vi "Test Initialize.vi"(0 "niDTS BT Rx Test in":refnum<class "niDTS BT Rx Test.lvclass">, 11 "error in (no error)":errorcluster) -> (4 "niDTS BT Rx Test out":refnum<class "niDTS BT Rx Test.lvclass">, 15 "error out":errorcluster)   [LabVIEW 2015, in "niDTS BT.lvlib" / "niDTS BT Rx Test.lvclass"]
uses:
  niDTS BT Rx Test.lvclass
  TestStand/TestStep/Objects/niDTS TestStep.lvclass
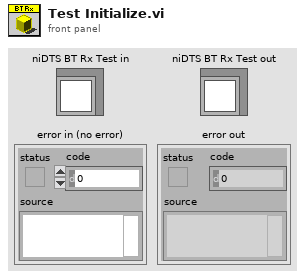
[diagram p1: front panel]
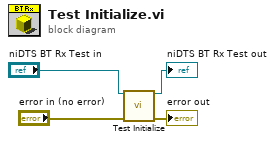
[diagram p0: block diagram]
diagram:
  n1 = call-parent "Test Initialize.vi"("niDTS TestStep in"="niDTS BT Rx Test in", "error in (no error)"="error in (no error)") -> ("niDTS TestStep out"=→"niDTS BT Rx Test out":refnum<class "niDTS BT Rx Test.lvclass">, "error out"=→"error out":errorcluster)  [unwired: 12 in]
